vi "UnbundleDir.vi"(0 "Direction":T1) -> (1 "Row":i32, 2 "Col":i32)   [LabVIEW 2017, in "Atom.lvclass"]
uses:
  Atom.lvclass
  Type Defs/Direction Enum.ctl
  Type Defs/SB Type Defs.lvlib
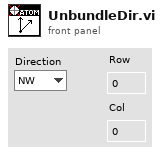
[diagram p1: front panel]
types:
  T1 = typedef "SB Type Defs.lvlib/Direction Enum.ctl" = enum16{"NW", "N", "NE", "E", "SE", "S", "SW", "W"}
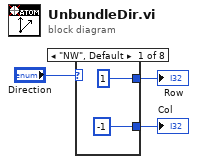
[diagram p0: block diagram]
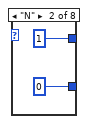
[diagram p2: hidden frame]
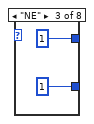
[diagram p3: hidden frame]
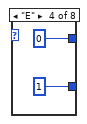
[diagram p4: hidden frame]
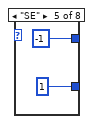
[diagram p5: hidden frame]
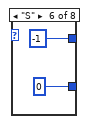
[diagram p6: hidden frame]
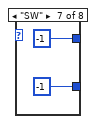
[diagram p7: hidden frame]
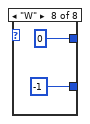
[diagram p8: hidden frame]
diagram:
  n1 = case shown="\"NW\", Default" "Direction" {
    tunnel: [1 ("Row") 1 ("Row") 1 ("Row") 0 ("Row") -1 ("Row") -1 ("Row") -1 ("Row") 0 ("Row")] -> w2
    tunnel: [-1 ("Row") 0 ("Row") 1 ("Row") 1 ("Row") 1 ("Row") 0 ("Row") -1 ("Row") -1 ("Row")] -> w1
    frame "NW", Default {
    }
    frame "N" {
    }
    frame "NE" {
    }
    frame "E" {
    }
    frame "SE" {
    }
    frame "S" {
    }
    frame "SW" {
    }
    frame "W" {
    }
  }
  "Row" <- w2
  "Col" <- w1
